vi "setDevices.vi"(8 "error in (no error)":errorcluster, 10 "Devices":T1[](array[typedef]), 11 "DAQmx in":refnum<class "DAQmx.lvclass">) -> (0 "error out":errorcluster, 3 "DAQmx out":refnum<class "DAQmx.lvclass">)   [LabVIEW 2019, in "DAQmx.lvclass"]
uses:
  DAQmx.lvclass
  typedefs/DeviceInfo--Cluster.ctl
  DAQmx.lvclass/DAQmx.ctl
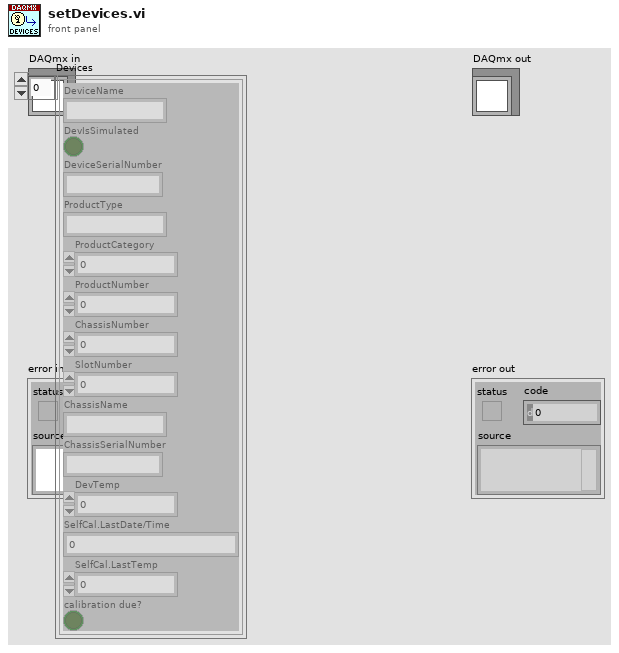
[diagram p1: front panel]
types:
  T1 = typedef "DAQmx.lvclass/DeviceInfo--Cluster.ctl" = cluster{"DeviceName":string, "DevIsSimulated":bool, "DeviceSerialNumber":string, "ProductType":string, "ProductCategory":i32, "ProductNumber":u32, "ChassisNumber":u32, "SlotNumber":u32, "ChassisName":string, "ChassisSerialNumber":string, "DevTemp":dbl, "SelfCal.LastDate/Time":string, "SelfCal.LastTemp":dbl, "calibration due?":bool}
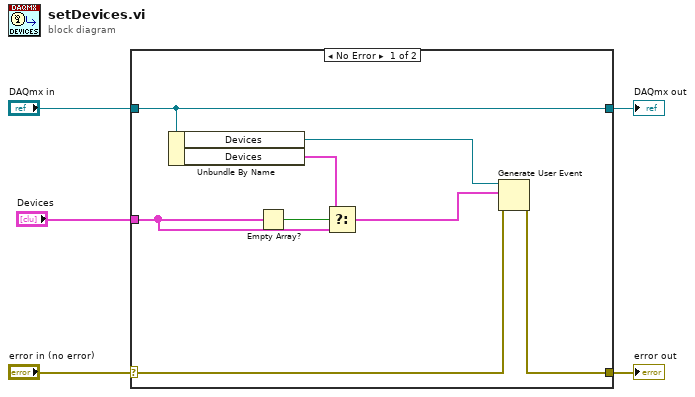
[diagram p0: block diagram]
diagram:
  n1 = case shown="No Error" "error in (no error)" {
    selector: "error in (no error)" -> [w11 w15]
    tunnel: [w10 w15] -> w4
    tunnel: [w13 w14] -> w2
    tunnel: "DAQmx in" -> [w13 w14]
    tunnel: "Devices" -> [w7 _]
    frame No Error {
      n2 = Unbundle By Name(w13) -> ("Devices"=w12:refnum<user-event>, "Devices"=w6:T1[])
      n3 = Empty Array?(array=w7) -> (empty?=w8:bool)
      n4 = Select(t=w6, s=w8, f=w7) -> (s? t:f=w9:T1[])
      n5 = Generate User Event(user event=w12, event data cluster=w9, error in=w11) -> (error out=w10:errorcluster)  [unwired: 1 in, 1 out]
    }
    frame Error {
    }
  }
  "error out" <- w4
  "DAQmx out" <- w2
